vi "CAN Initialize.vi"(10 "Btr0Btr1":u16=28 format="%.0x", 11 "Channel":u16=81 format="%.0x") -> (2 "Channel out":u16, 3 "function return":u32 format="%.0x")   [LabVIEW 2020, in "PCANBasic.lvlib"]
doc: "TPCANStatus __stdcall CAN_Initialize(\n TPCANHandle Channel, \n TPCANBaudrate Btr0Btr1, \n TPCANType HwType _DEF_ARG,\n DWORD IOPort _DEF_ARG, \n WORD Interrupt _DEF_ARG);"
uses:
  PCANBasic.lvlib
  <userlib>/PCANBasic/PCANBasic.dll
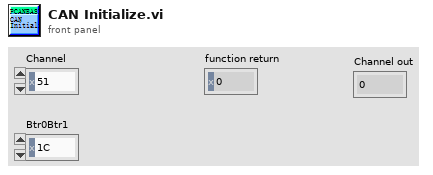
[diagram p1: front panel]
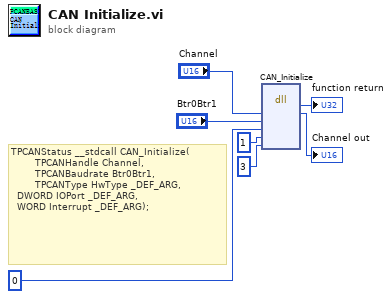
[diagram p0: block diagram]
diagram:
  # "TPCANStatus __stdcall CAN_Initialize(\n        TPCANHandle Channel, \n        TPCANBaudrate Btr0Btr1, \n        TPCANType HwType _DEF_ARG,\n\t\tDWORD IOPort _DEF_ARG, \n\t\tWORD Interrupt _DEF_ARG);"
  n1 = dll-call lib="D:/Program Files (x86)/National Instruments/LabVIEW 2020/user.lib/PCANBasic/PCANBasic.*" fn="CAN_Initialize"("Channel"="Channel", "Btr0Btr1"="Btr0Btr1", "TPCANtype"=u8 0, "IOport"=u32 1, "interrupt"=u16 3) -> ("返回类型"=→"function return":u32, "Channel"=→"Channel out":u16)  [unwired: 7 in, 2 out]
